vi "3D_Lab_v1.0.vi"() -> ()   [LabVIEW 2018]
uses:
  <vilib>/Native 3D Graph/xcontrol/3DPC_SurfacePlot.xctl
panel:
  out "3D Graph":refnum<class "Base Datatype.lvclass">[](xcontrol)
  out "element":dbl
  out "element 3":dbl
  out "element 2":dbl format="%#.8g"
  out "array":dbl[][](array[numeric])
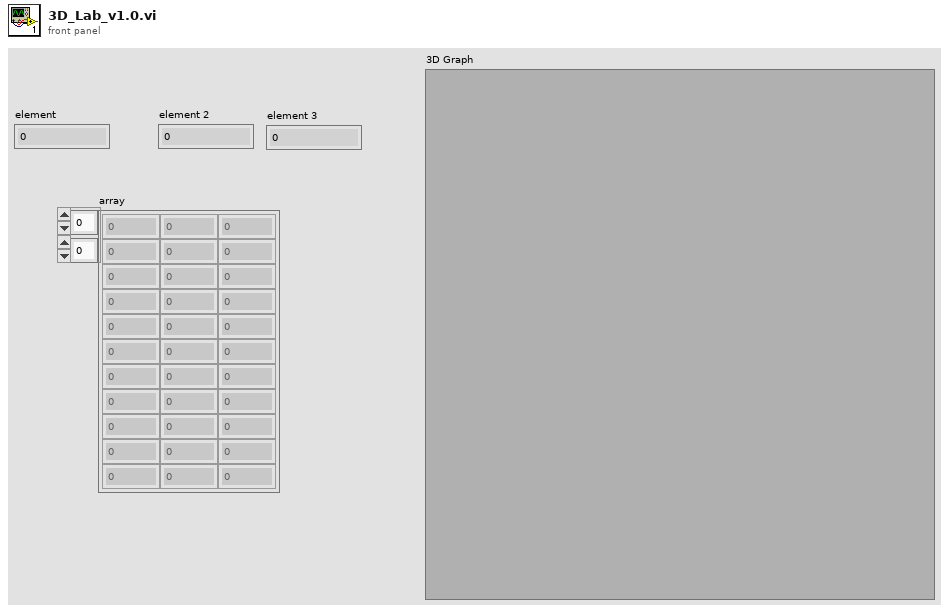
[diagram p1: front panel]
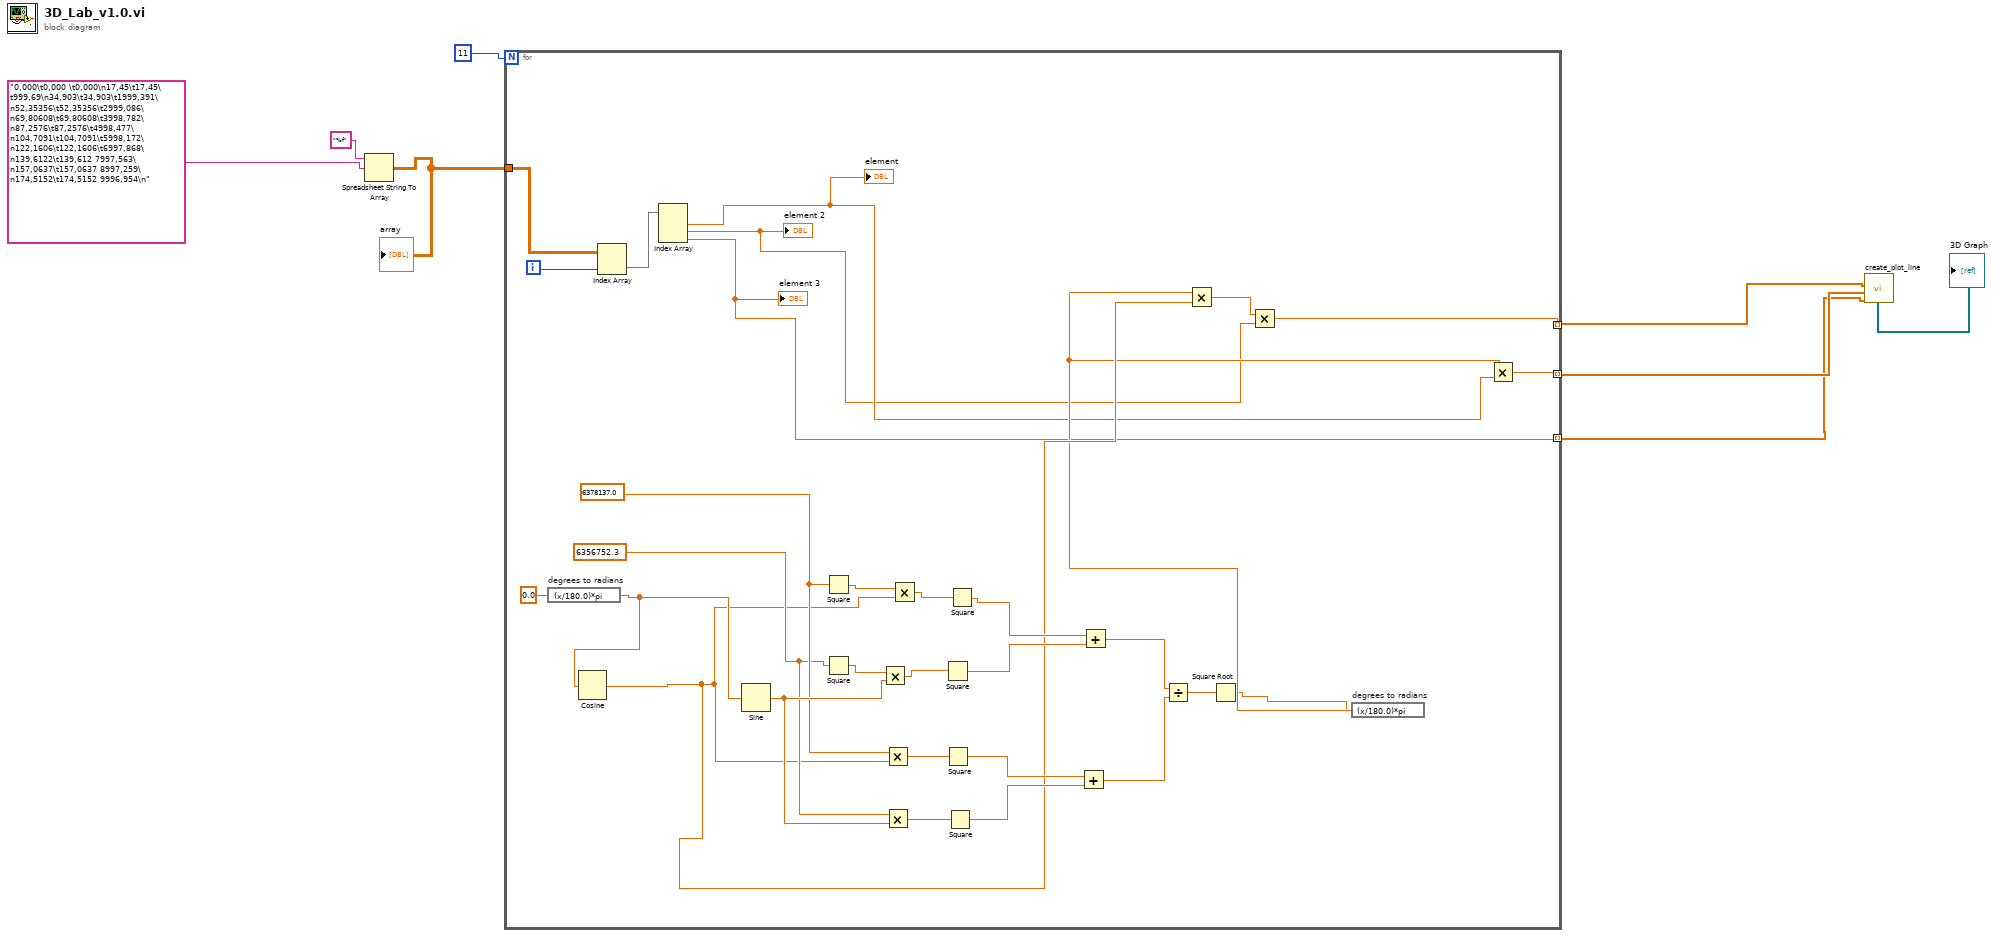
[diagram p0: block diagram]
diagram:
  n1 = Spreadsheet String To Array(format string="%f", spreadsheet string="0,000\t0,000 \t0,000\n17,45\t17,45\t999,69\n34,903\t34,903\t1999,391\n52,35356\t52,35356\t2999,086\n69,80608\t69,80608\t3998,782\n87,2576\t87,2576\t4998,477\n104,7091\t104,7091\t5998,172\n122,1606\t122,1606\t6997,868\n139,6122\t139,612 7997,563\n157,0637\t157,0637 8997,259\n174,5152\t174,5152 9996,954\n") -> (array=w6:dbl[][])  [unwired: 2 in]
  "array" <- w6
  n2 = for {
    N: 11 -> [_]
    tunnel: w6 -> [w36]
    tunnel: [w15] -> w3 mode=indexing
    tunnel: [w14] -> w2 mode=indexing
    tunnel: [w10] -> w1 mode=indexing
    i -> [w38]
    w23 = 6378137.0
    w20 = 6356752.3
    n3 = expression code="(x/180.0)*pi" "degrees to radians"(0.0) -> (w25:dbl)
    n4 = Cosine(x=w25) -> (cos(x)=w18:dbl)
    n5 = Index Array(array=w36, index (row)=w38) -> (element=w37:dbl[])  [unwired: 1 in]
    n6 = Index Array(array=w37) -> (element #1=w12:dbl, element #2=w11:dbl, element #3=w10:dbl)  [unwired: 3 in]
    "element 2" <- w11
    "element 3" <- w10
    "element" <- w12
    n7 = Sine(x=w25) -> (sin(x)=w32:dbl)
    n8 = Square(x=w23) -> (x^2=w24:dbl)
    n9 = Square(x=w20) -> (x^2=w19:dbl)
    n10 = Multiply(x=w19, y=w32) -> (x*y=w35:dbl)
    n11 = Multiply(x=w23, y=w18) -> (x*y=w33:dbl)
    n12 = Multiply(x=w20, y=w32) -> (x*y=w31:dbl)
    n13 = Multiply(x=w24, y=w18) -> (x*y=w22:dbl)
    n14 = Square(x=w35) -> (x^2=w34:dbl)
    n15 = Square(x=w33) -> (x^2=w30:dbl)
    n16 = Square(x=w31) -> (x^2=w29:dbl)
    n17 = Square(x=w22) -> (x^2=w21:dbl)
    n18 = Add(x=w30, y=w29) -> (x+y=w27:dbl)
    n19 = Add(x=w21, y=w34) -> (x+y=w28:dbl)
    n20 = Divide(x=w28, y=w27) -> (x/y=w26:dbl)
    n21 = Square Root(x=w26) -> (sqrt(x)=w9:dbl)
    n22 = expression code="(x/180.0)*pi" "degrees to radians"(w9) -> (w16:dbl)
    n23 = Multiply(x=w16, y=w18) -> (x*y=w17:dbl)
    n24 = Multiply(x=w17, y=w11) -> (x*y=w15:dbl)
    n25 = Multiply(x=w16, y=w12) -> (x*y=w14:dbl)
  }
  n26 = call <vilib>:"create_plot_line.vi"("z vector"=w1, "y vector"=w2, "x vector"=w3) -> ("plots out"=→"3D Graph":refnum<class "Base Datatype.lvclass">[])  [unwired: 2 in, 6 out]
